vi "Incomming Array Handler.vi"(3 "Array":dbl[](array[numeric])) -> ()   [LabVIEW 2016]
uses:
  Typedef/MCU_addresses.ctl
panel:
  out "Array 3":dbl[](array[numeric])
  out "Array 2":dbl[](array[numeric])
  out "error out 3":errorcluster
  out "element":dbl
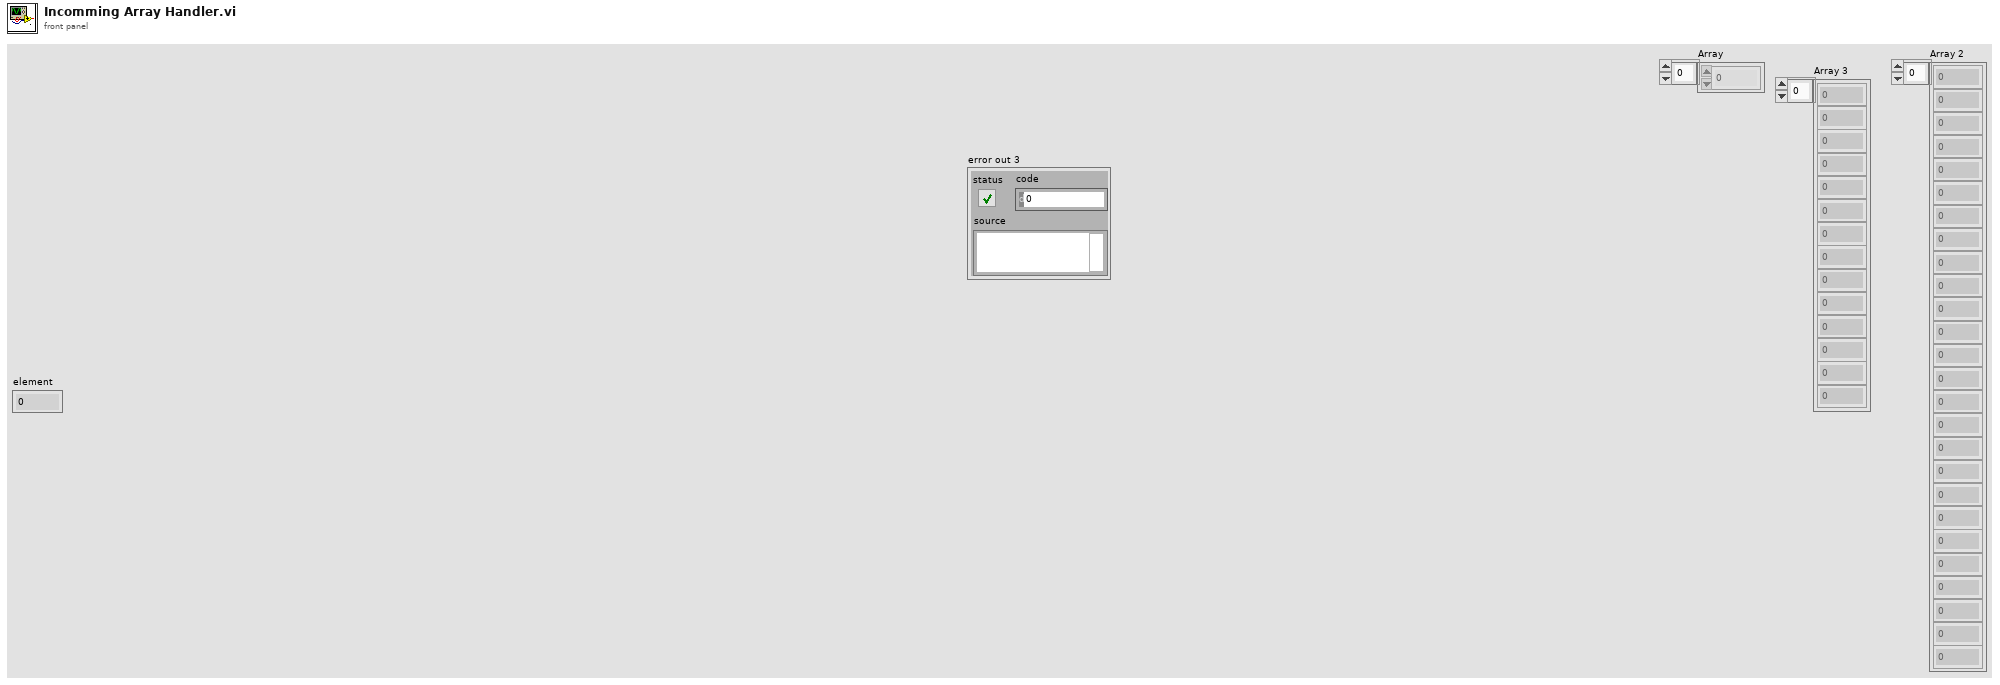
[diagram p1: front panel]
types:
  T1 = typedef "MCU_addresses.ctl" = string
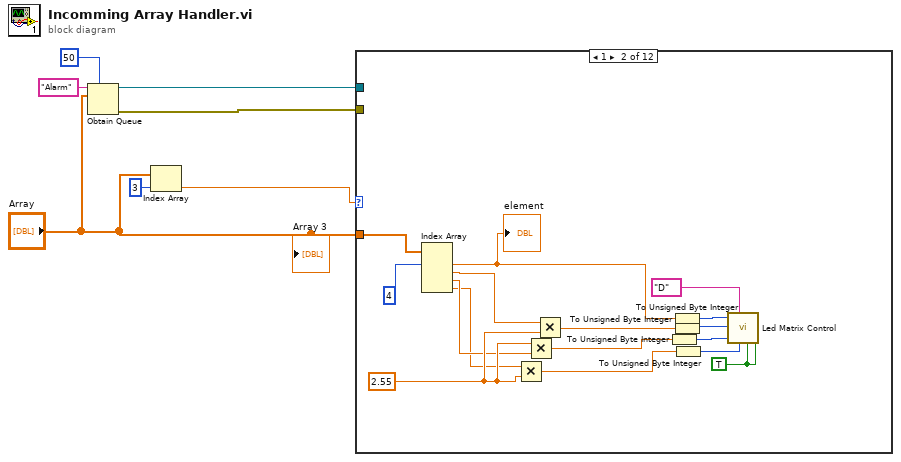
[diagram p0: block diagram]
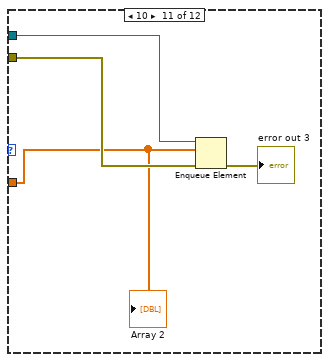
[diagram p11: hidden frame]
diagram:
  n1 = Obtain Queue(max queue size (-1, unlimited)=50, name (unnamed)="Alarm", element data type="Array") -> (queue out=w4:refnum<queue>, error out=w5:errorcluster)  [unwired: 2 in, 1 out]
  n2 = Index Array(array="Array", index=3) -> (element=w6:dbl)
  n3 = case shown="1" w6 {
    tunnel: "Array" -> [_ w18 _ _ _ _ _ _ _ _ w24 _]
    tunnel: w5 -> [_ _ _ _ _ _ _ _ _ _ w26 _]
    tunnel: w4 -> [_ _ _ _ _ _ _ _ _ _ w25 _]
    frame 0, Default {
    }
    frame 1 {
      w17 = TRUE ("Close Tab")
      w22 = 2.55
      n4 = Index Array(array=w18, index #1=4 ("length")) -> (element #1=w11:dbl, element #2=w21:dbl, element #3=w20:dbl, element #4=w19:dbl)  [unwired: 3 in]
      "element" <- w11
      n5 = Multiply(x=w19, y=w22) -> (x*y=w8:dbl)
      n6 = Multiply(x=w22, y=w20) -> (x*y=w9:dbl)
      n7 = Multiply(x=w21, y=w22) -> (x*y=w10:dbl)
      n8 = To Unsigned Byte Integer(number=w9) -> (unsigned 8bit integer=w15:u8)
      n9 = To Unsigned Byte Integer(number=w11) -> (unsigned 8bit integer=w13:u8)
      n10 = To Unsigned Byte Integer(number=w10) -> (unsigned 8bit integer=w14:u8)
      n11 = To Unsigned Byte Integer(number=w8) -> (unsigned 8bit integer=w16:u8)
      n12 = call "Led Matrix Control.vi"("LED Location"=w13, "MCU addresses"=T1 "D", "Red"=w14, "Green"=w15, "Blue"=w16, "Send To MCU"=w17, "Close Tab"=w17) -> ()  [unwired: 2 in, 1 out]
    }
    frame 2 {
    }
    frame 3 {
    }
    frame 4 {
    }
    frame 5 {
    }
    frame 6 {
    }
    frame 7 {
    }
    frame 8 {
    }
    frame 9 {
    }
    frame 10 {
      n13 = Enqueue Element(queue=w25, element=w24, error in (no error)=w26) -> (error out=→"error out 3":errorcluster)  [unwired: 1 in, 2 out]
      "Array 2" <- w24
    }
    frame 11 {
    }
  }
  "Array 3" <- "Array"
